vi "Stop Core.vi"(10 "final error code":i32, 11 "Generic Optimization in":refnum<class "Generic Optimization.lvclass">) -> (3 "Generic Optimization out":refnum<class "Generic Optimization.lvclass">)   [LabVIEW 2018, in "Generic Optimization Actor.lvlib" / "Generic Optimization.lvclass"]
doc: "(<B>Filename</B>: Actor Framework.lvlib:Actor.lvclass:Stop Core.vi)\n\nDefines what the actor does before it stops. Use the <B>final error code</B> input to determine whether the actor shut down in response to an error.\n\nBy default, this method does nothing. A descendant class may override it to define behavior, such as shutting down any processes the actor initiated in its override of the Actor Core method."
uses:
  Generic Optimization.lvclass
  <vilib>/ActorFramework/Time-Delayed Send Message/Time-Delay Override Options.ctl
  Generic Optimization.lvclass/Generic Optimization.ctl
  Device Communication and Control Abstract Actor/Device Communication and Control Abstract/Device Communication and Control Abstract.lvclass
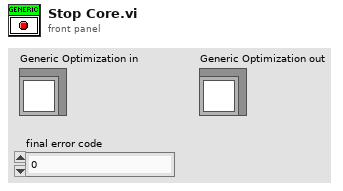
[diagram p1: front panel]
types:
  T1 = typedef "Time-Delay Override Options.ctl" = enum16{"Send next copy now", "Skip next scheduled copy", "Send next copy now and stop all further copies", "Stop all further copies"}
  T2 = typedef "Generic Optimization Actor.lvlib/Generic Optimization.lvclass/Delivery Notifiers.ctl" = cluster{"watchdogReset":refnum<notifier>, "Find and Rejoin":refnum<notifier>}
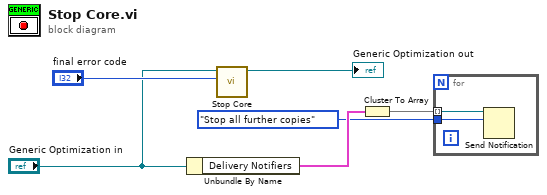
[diagram p0: block diagram]
diagram:
  n1 = Unbundle By Name("Generic Optimization in") -> ("Delivery Notifiers"=w3:T2)
  n2 = call-parent "Stop Core.vi"("final error code"="final error code", "EMS Generic in"="Generic Optimization in") -> ("EMS Generic out"=→"Generic Optimization out":refnum<class "Generic Optimization.lvclass">)  [unwired: 9 in]
  n3 = Cluster To Array(cluster=w3) -> (array=w1:refnum<notifier>[])
  n4 = for {
    tunnel: Time-Delay_Override_Options."Stop all further copies" ("notification") -> [w8]
    tunnel: w1 -> [w7] mode=indexing
    n5 = Send Notification(notification=w8, notifier=w7) -> ()  [unwired: 1 in, 2 out]
  }
